vi "HP34401-n-meas.vi"(2 "Tc":sgl=1.0 format="%.2f", 3 "N":i32=5 min=1 max=500, 4 "Function (0:V DC)":u16(ring) items=["DC Voltage", "AC Voltage", "2--Wire Resistance", "4-Wire Resistance", "DC Current", "AC Current", "Frequency", "Period", "Continuity", "Diode Checking", "VDC: VDC Ratio"]) -> (0 "error out":errorcluster, 1 "Vet out":dbl[](array[numeric]) format="%.2f")   [LabVIEW 2012]
doc: "M. Ferrari M. Corti 2004\nMisura Ripetuta Vdc con HP34401A e DRV"
uses:
  <instrlib>/Agilent 34401/Public/Data/Read (Multiple Points).vi
  <instrlib>/Agilent 34401/Agilent 34401.lvlib
panel:
  in  "VISA resource name":refnum<visa-resource-name>
  # "MISURE RIPETUTE CON MULTIMETRO HP34401A ed USO dei VI del DRIVER di LabVIEW \n    Realizzare un VI che svolga le seguenti funzioni: \n   - configura il multimetro per una misura di tensione su un segnale sinusoidale in autoscala \n   - ripete la misura per un numero N (N=<100) di volte ad intervalli di tempo Tc, selezionabili da pannello\n   - memorizza i dati ottenuti in un vettore e segnala errori eventuali"
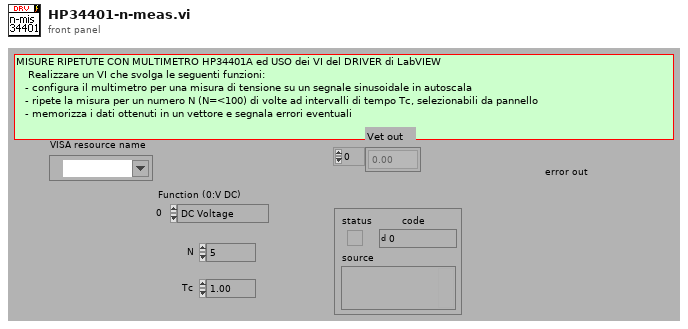
[diagram p1: front panel]
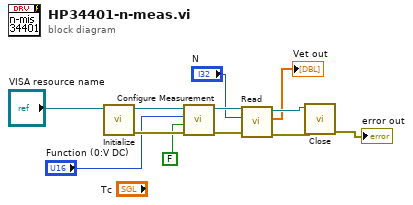
[diagram p0: block diagram]
diagram:
  n1 = call <instrlib>:"Initialize.vi"("VISA resource name"="VISA resource name") -> ("error out"=w11:errorcluster, "VISA resource name out"=w12:refnum<visa-resource-name>)  [unwired: 9 in]
  n2 = call <instrlib>:"Configure Measurement.vi"("error in (no error)"=w11, "Enable Auto Range (T: Enable)"=FALSE ("Range/Resolution (T:Auto)"), "Function (0: DC Voltage)"="Function (0:V DC)", "VISA resource name"=w12) -> ("error out"=w6:errorcluster, "VISA resource name out"=w4:refnum<visa-resource-name>)  [unwired: 6 in]
  n3 = call-poly <instrlib>:"Read.vi"("error in (no error)"=w6, "Sample Count (1)"="N", "VISA resource name"=w4) -> ("error out"=w5:errorcluster, "Measurements"=→"Vet out":dbl[], "VISA resource name out"=w3:refnum<visa-resource-name>)  [unwired: 6 in]
  n4 = call <instrlib>:"Close.vi"("error in (no error)"=w5, "VISA resource name"=w3) -> ("error out"=→"error out":errorcluster)  [unwired: 9 in]
